vi "Run Rx - New Data.vi"(6 "New Data Option":T1, 7 "Packet Count in":dbl, 8 "error in (no error)":errorcluster, 10 "New Data":bool, 11 "New Data Ref":T2) -> (0 "error out":errorcluster, 5 "Packet Count out":dbl)   [LabVIEW 2016, in "UDP-Custom-Device Engine.lvlib"]
uses:
  UDP-Custom-Device Engine.lvlib
  <vilib>/NI/NIVS Inline Async API/_Data Access Engine/Data Access Engine/Types/Write.DVR.ctl
  <vilib>/NI/NIVS Inline Async API/_Data Access Engine/Access Type Classes/Write/Write.lvclass
  Shared/Types/Shared - New Data Options.ctl
  <vilib>/NI/NIVS Inline Async API/_Data Access Engine/Access Type Classes/Write/Write.lvclass/Write.ctl
  <vilib>/NI/NIVS Inline Async API/_Data Access Engine/Data Access Engine/Methods/Write.Data.vi
  <vilib>/NI/NIVS Inline Async API/_Data Access Engine/Access Type Classes/Write/Write.ProcessData.vi
  <vilib>/NI/NIVS Inline Async API/_Data Access Engine/Data Access Engine/Data Access Engine.lvclass
  Shared/UDP-Custom-Device Shared.lvlib
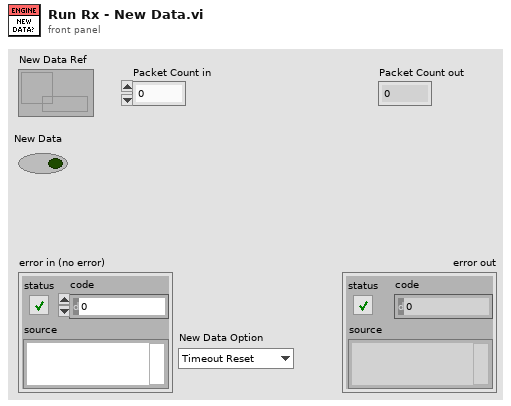
[diagram p1: front panel]
types:
  T1 = typedef "UDP-Custom-Device Shared.lvlib/Shared - New Data Options.ctl" = enum16{"Timeout Reset", "Counter"}
  T2 = typedef "Data Access Engine.lvlib/Data Access Engine.lvclass/Write.DVR.ctl" = refnum<data-value>
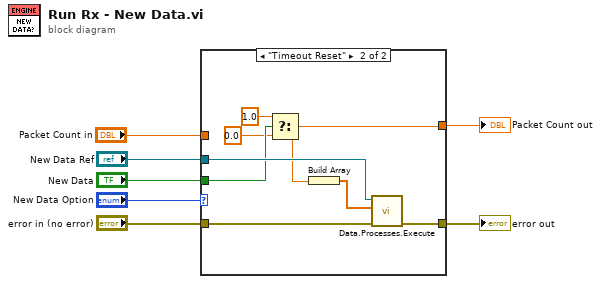
[diagram p0: block diagram]
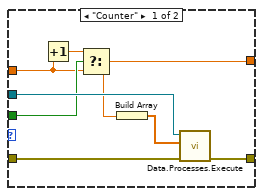
[diagram p2: hidden frame]
diagram:
  n1 = case shown="\"Timeout Reset\"" "New Data Option" {
    tunnel: "error in (no error)" -> [w14 w22]
    tunnel: [w13 w21] -> w6
    tunnel: "New Data Ref" -> [w12 w20]
    tunnel: "New Data" -> [w11 w19]
    tunnel: [w9 w18] -> w3
    tunnel: "Packet Count in" -> [w8 _]
    frame "Counter" {
      n2 = Increment(x=w8) -> (x+1=w10:dbl)
      n3 = Select(t=w10, s=w11, f=w8) -> (s? t:f=w9:dbl)
      n4 = Build Array(w9) -> (w15:dbl[])
      n5 = call-poly <vilib>:"Data.Processes.Execute.vi"("error in (no error)"=w14, "Values"=w15, "Ref"=w12) -> ("error out"=w13:errorcluster)  [unwired: 8 in]
    }
    frame "Timeout Reset" {
      n6 = Select(t=1.0 ("Packet Count in"), s=w19, f=0.0 ("Packet Count in")) -> (s? t:f=w18:dbl)
      n7 = Build Array(w18) -> (w23:dbl[])
      n8 = call-poly <vilib>:"Data.Processes.Execute.vi"("error in (no error)"=w22, "Values"=w23, "Ref"=w20) -> ("error out"=w21:errorcluster)  [unwired: 8 in]
    }
  }
  "error out" <- w6
  "Packet Count out" <- w3
